vi "2-2 用公式法计算x阶层和.vi"() -> ()   [LabVIEW 2019]
panel:
  out "y":i32
  in  "x":dbl
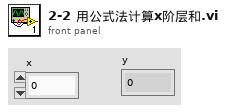
[diagram p1: front panel]
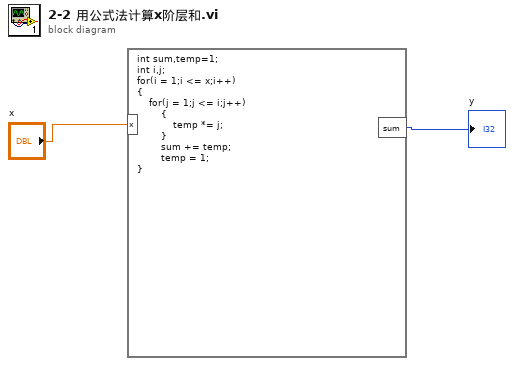
[diagram p0: block diagram]
diagram:
  n1 = formula code="int sum,temp=1;\nint i,j;\nfor(i = 1;i <= x;i++)\n{\n    for(j = 1;j <= i;j++)\n        {\n            temp *= j;\n        }\n        sum += temp;\n        temp = 1;\n}"("x"="x") -> ("sum"=→"y":i32)
